vi "Laser_Control_1D.vi"() -> ()   [LabVIEW 2022 SP3]
uses:
  ADAM Client/Sub VIs/ADAM Controls/Update_scan_value.ctl
  Fibre_Flow_Mode.ctl
panel:
  out "GetMaxPower (mW)":dbl
  in  "stop":bool
  out "Loop No":i32
  in  "Power (mW)":dbl
  in  "Mode":T1
  out "error out":errorcluster
  in  "BSALaserCtrl.IBSALaser 2":refnum<k7>
  out "Status":string[](array[string])
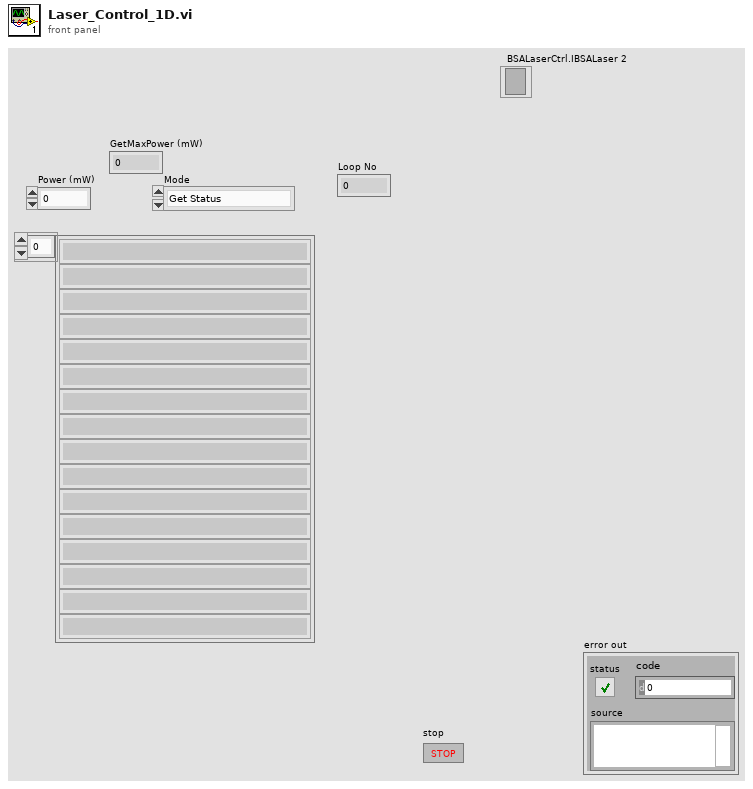
[diagram p1: front panel]
types:
  T1 = typedef "Fibre_Flow_Mode.ctl" = enum16{"Get Status", "Set Power", "Turn Laser On", "Turn Laser Off", "Shutter Open", "Shutter Closed", "Attenuated", "Disconnect"}
  T2 = typedef "Update_scan_value.ctl" = cluster{"Channel Name":string, "New Value":dbl, "!Auto_Off":bool}
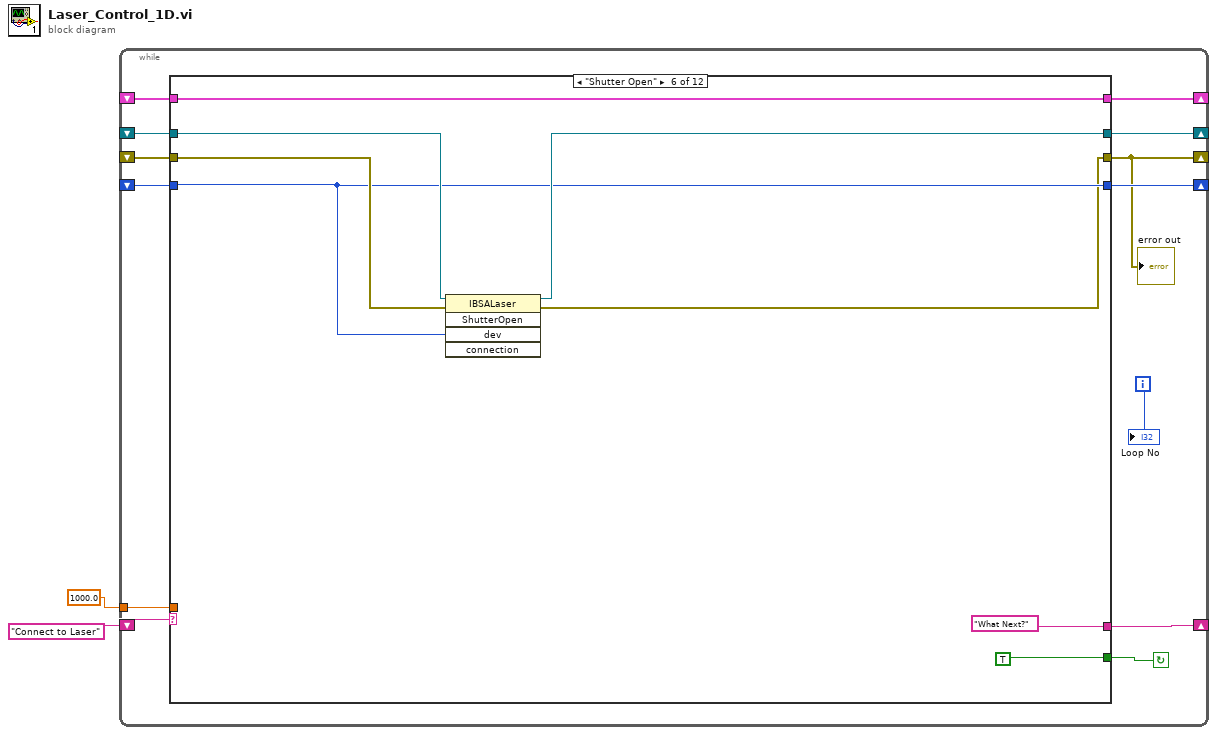
[diagram p0: block diagram]
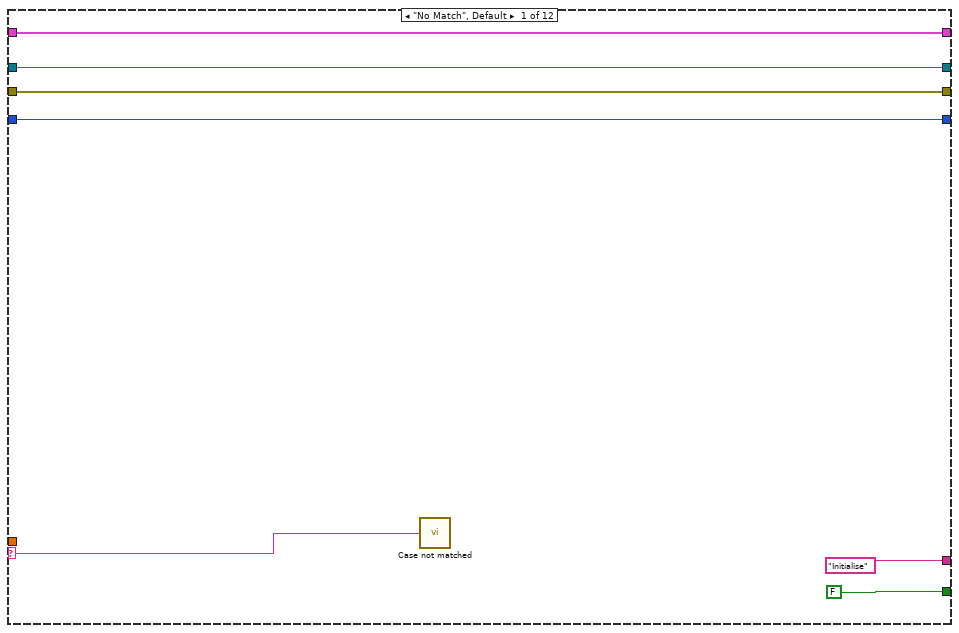
[diagram p2: hidden frame]
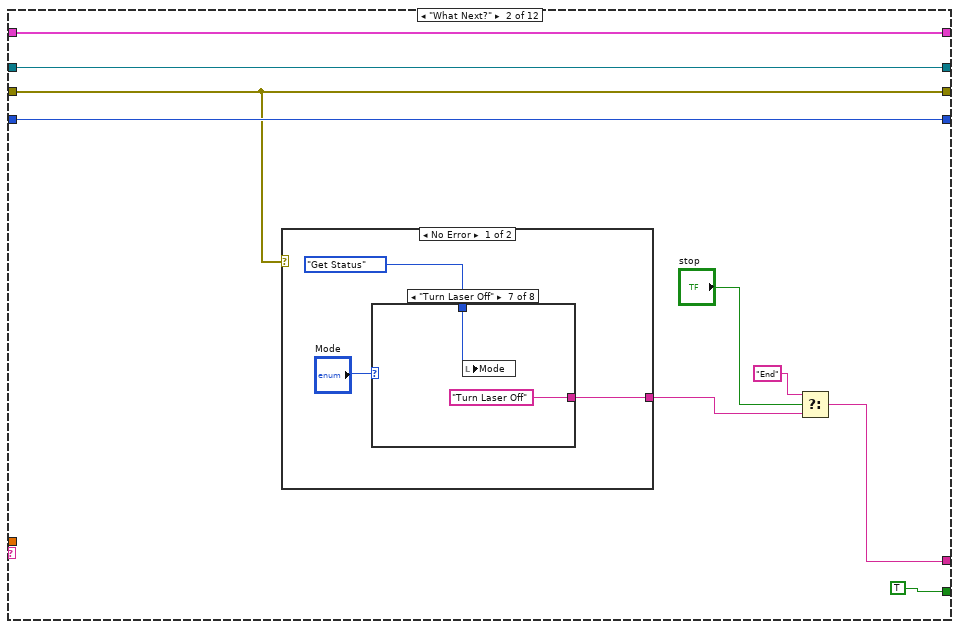
[diagram p3: hidden frame]
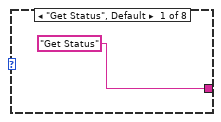
[diagram p4: hidden frame]
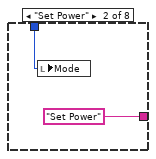
[diagram p5: hidden frame]
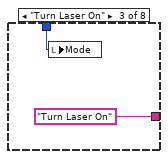
[diagram p6: hidden frame]
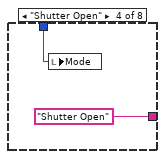
[diagram p7: hidden frame]
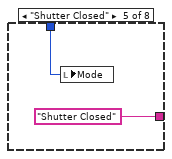
[diagram p8: hidden frame]
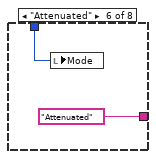
[diagram p9: hidden frame]
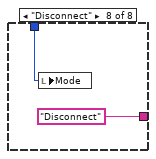
[diagram p10: hidden frame]
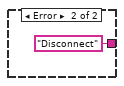
[diagram p11: hidden frame]
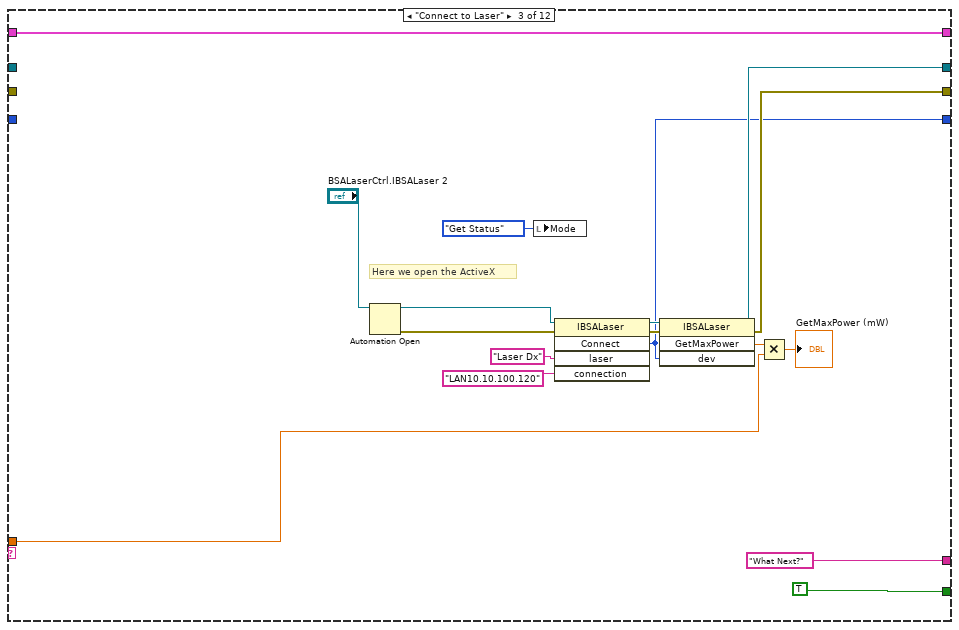
[diagram p12: hidden frame]
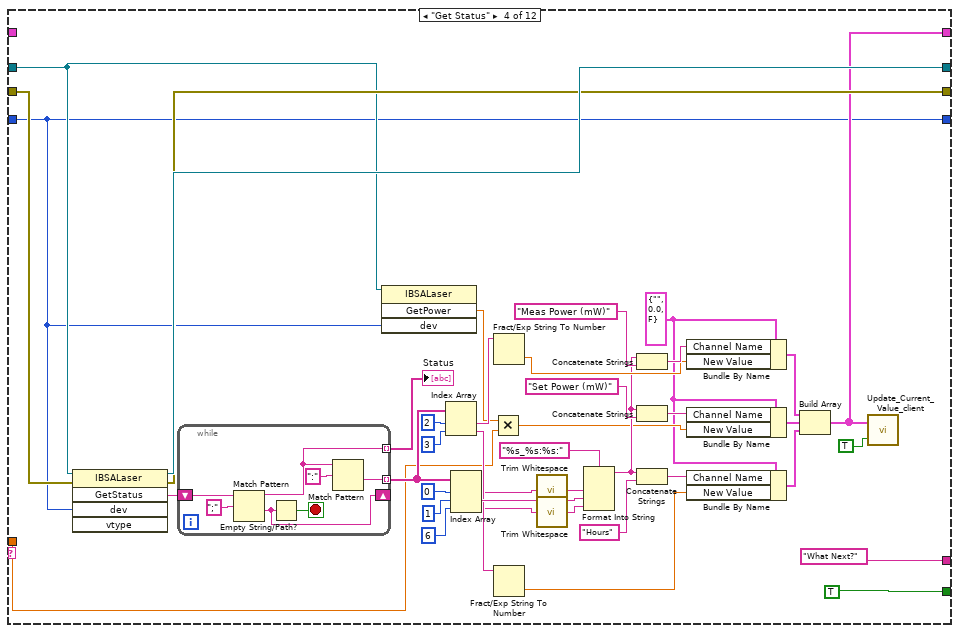
[diagram p13: hidden frame]
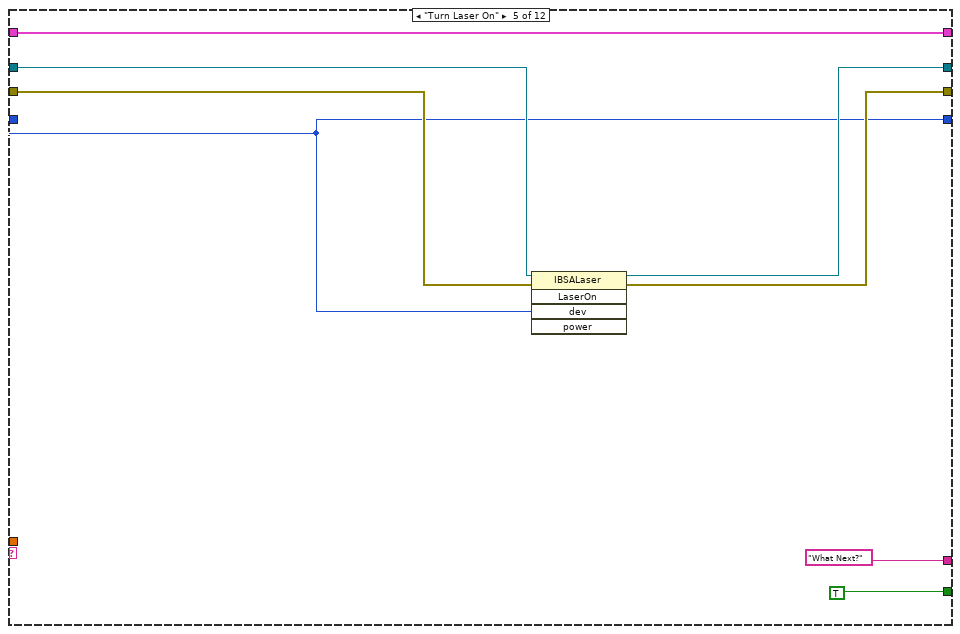
[diagram p14: hidden frame]
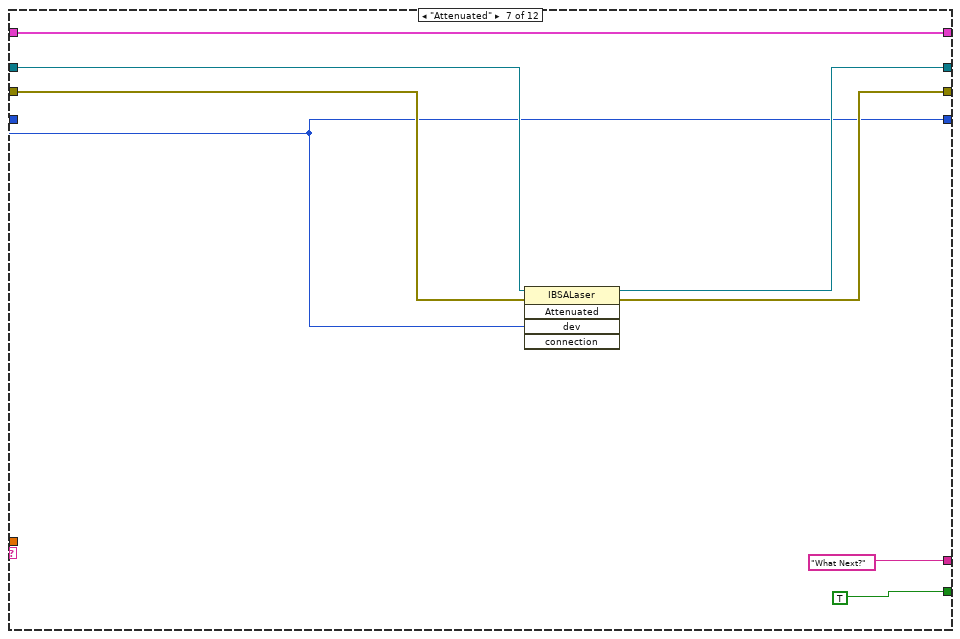
[diagram p15: hidden frame]
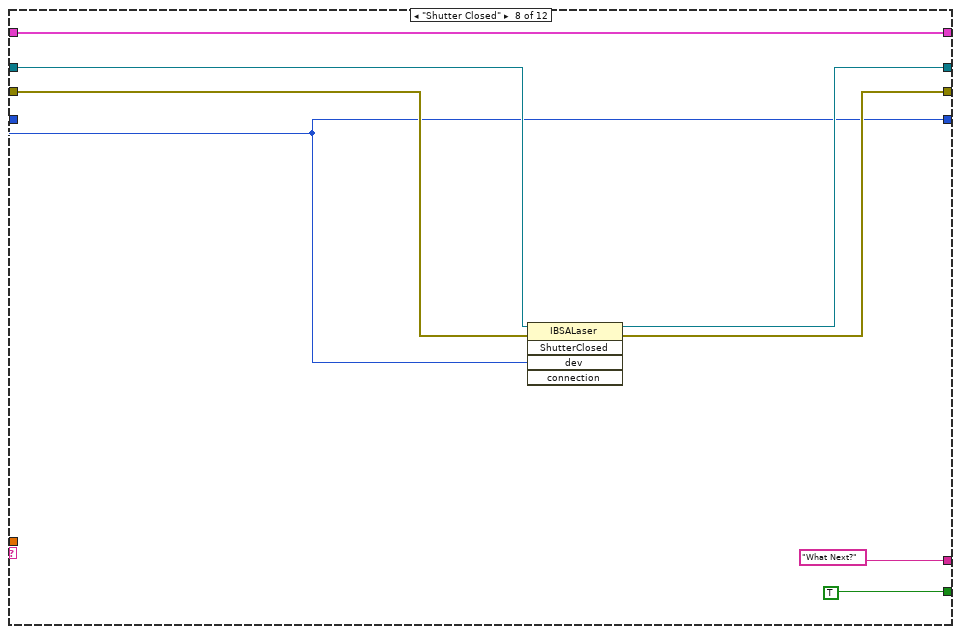
[diagram p16: hidden frame]
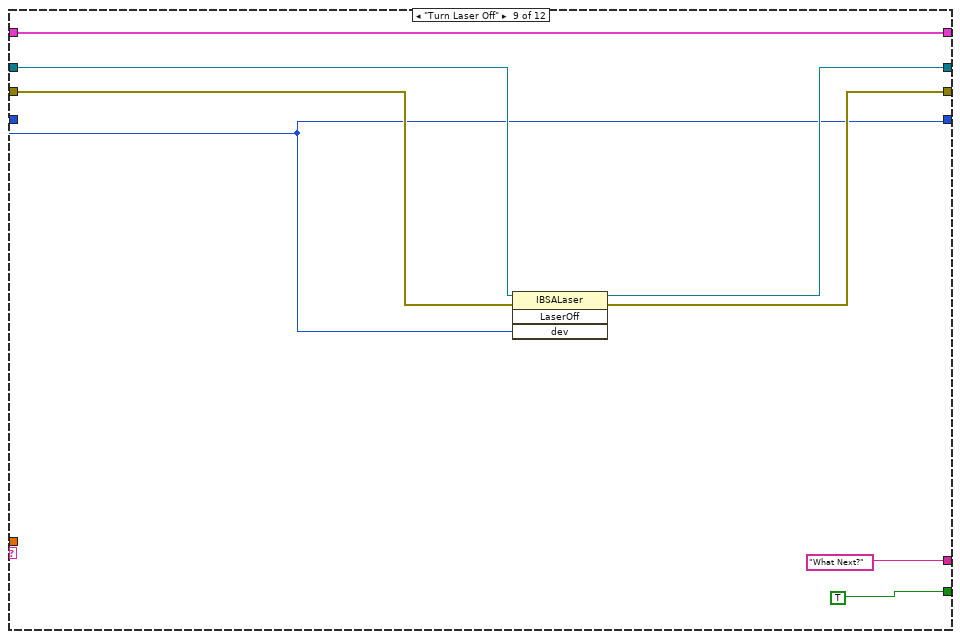
[diagram p17: hidden frame]
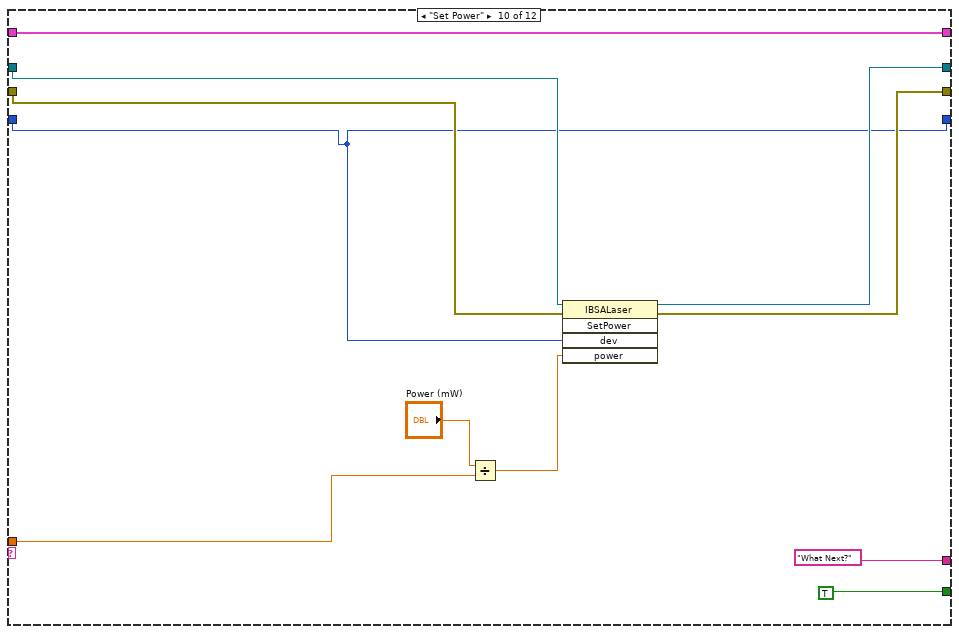
[diagram p18: hidden frame]
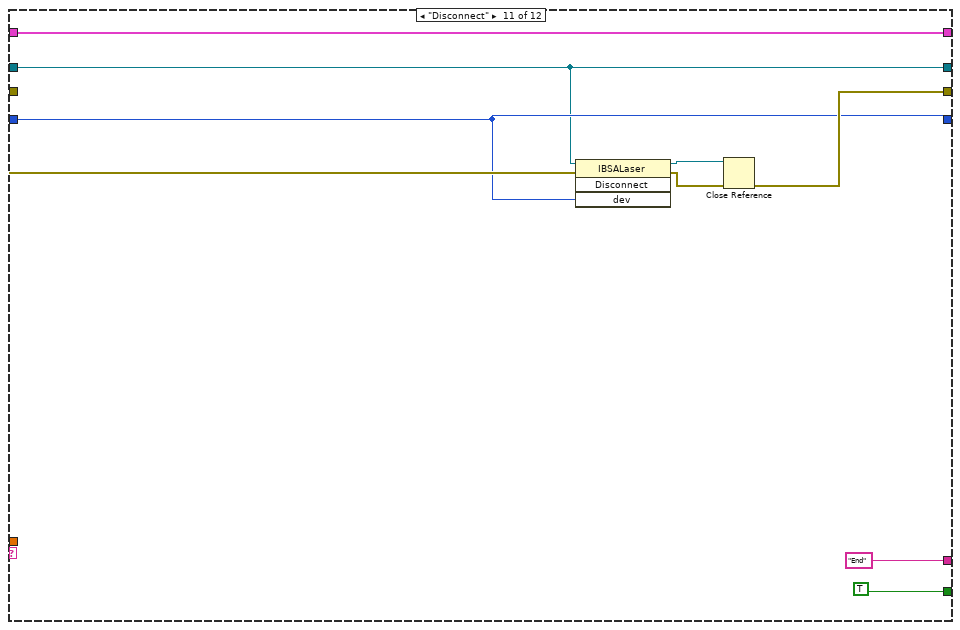
[diagram p19: hidden frame]
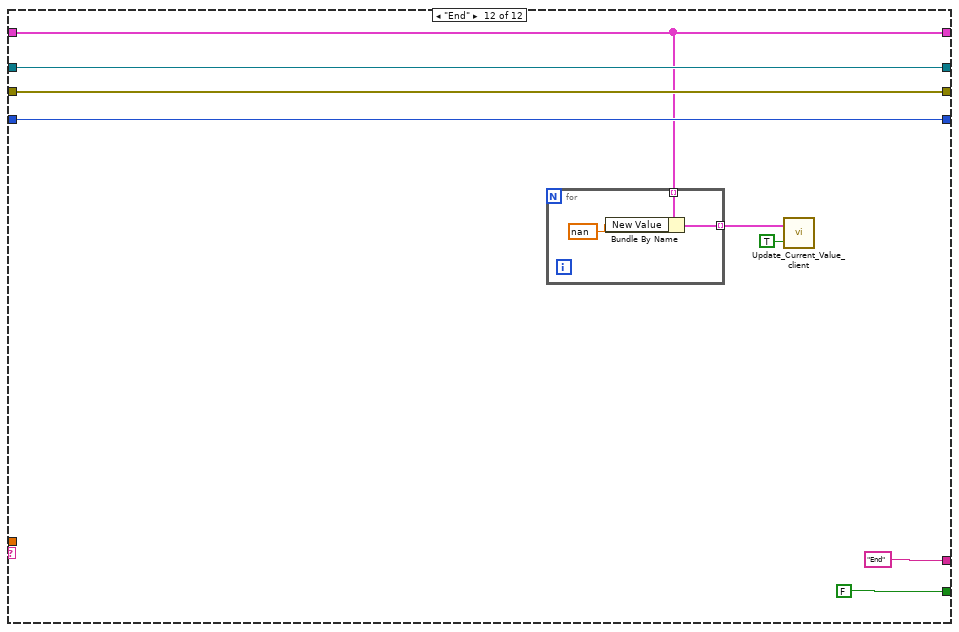
[diagram p20: hidden frame]
diagram:
  n1 = while {
    shift-left: "Connect to Laser" -> [w13]
    shift-right: [w14] -> _
    shift-right: [w12] -> _
    shift-left: _ -> [w10]
    shift-right: [w7] -> _
    shift-left: _ -> [w9]
    shift-right: [w11] -> _
    shift-left: _ -> [w8]
    shift-right: [w5] -> _
    shift-left: _ -> [w4]
    tunnel: 1000.0 ("y") -> [w3]
    i -> [w6]
    stop <- w15 continue-if-true
    n2 = case shown="\"Shutter Open\"" w13 {
      selector: w13 -> [w20 _ _ _ _ _ _ _ _ _ _ _]
      tunnel: [FALSE TRUE TRUE TRUE TRUE TRUE TRUE TRUE TRUE TRUE TRUE FALSE] -> w15
      tunnel: ["Initialise" w24 "What Next?" "What Next?" "What Next?" "What Next?" "What Next?" "What Next?" "What Next?" "What Next?" "End" "End"] -> w14
      tunnel: [w19 w31 w57 w104 w119 w127 w135 w143 w151 w162 w168 w180] -> w12
      tunnel: [w18 w29 w56 w103 w118 w124 w134 w142 w150 w161 w170 w179] -> w7
      tunnel: [w17 w30 w55 w78 w117 w126 w133 w141 w149 w160 w169 w181] -> w11
      tunnel: w10 -> [w19 w31 _ w79 w121 w129 w137 w145 w153 w164 w168 w180]
      tunnel: w9 -> [w18 w29 _ w105 w120 w128 w136 w144 w152 w163 w171 w179]
      tunnel: w8 -> [w17 w30 _ w78 w117 w126 w133 w141 w149 w160 w169 w181]
      tunnel: [w16 w28 w60 w80 w116 w125 w132 w140 w148 w159 w167 w177] -> w5
      tunnel: w4 -> [w16 w28 w60 _ w116 w125 w132 w140 w148 w159 w167 w177]
      tunnel: w3 -> [_ _ w52 w71 _ _ _ _ _ w157 _ _]
      frame "No Match", Default {
        n3 = call "Case not matched.vi"("Case Name not Matched"=w20) -> ()
      }
      frame "What Next?" {
        n4 = case shown="No Error" w29 {
          tunnel: [w33 "Disconnect"] -> w25
          frame No Error {
            n5 = case shown="\"Turn Laser Off\"" "Mode" {
              tunnel: ["Get Status" "Set Power" "Turn Laser On" "Shutter Open" "Shutter Closed" "Attenuated" "Turn Laser Off" "Disconnect"] -> w33
              tunnel: Fibre_Flow_Mode."Get Status" ("Mode") -> [_ w36 w38 w40 w42 w44 w46 w48]
              frame "Get Status", Default {
              }
              frame "Set Power" {
                n6 = local write "Mode"(w36) -> ()
              }
              frame "Turn Laser On" {
                n7 = local write "Mode"(w38) -> ()
              }
              frame "Shutter Open" {
                n8 = local write "Mode"(w40) -> ()
              }
              frame "Shutter Closed" {
                n9 = local write "Mode"(w42) -> ()
              }
              frame "Attenuated" {
                n10 = local write "Mode"(w44) -> ()
              }
              frame "Turn Laser Off" {
                n11 = local write "Mode"(w46) -> ()
              }
              frame "Disconnect" {
                n12 = local write "Mode"(w48) -> ()
              }
            }
          }
          frame Error {
          }
        }
        n13 = Select(t="End", s="stop", f=w25) -> (s? t:f=w24:string)
      }
      frame "Connect to Laser" {
        # "Here we open the ActiveX"
        n14 = Automation Open(Automation Refnum="BSALaserCtrl.IBSALaser 2") -> (Automation Refnum=w63:refnum<k7>, error out=w64:errorcluster)  [unwired: 3 in]
        n15 = local write "Mode"(Fibre_Flow_Mode."Get Status" ("Mode")) -> ()
        n16 = invoke class="IBSALaser" method="Connect"(reference=w63, error in=w64, "laser"="Laser Dx", "connection"="LAN10.10.100.120") -> (reference out=w59:refnum<k7>, error out=w58:errorcluster, "Connect"=w55:i64)  [unwired: 1 in, 2 out]
        n17 = invoke class="IBSALaser" method="GetMaxPower"(reference=w59, error in=w58, "dev"=w55) -> (reference out=w57:refnum<k7>, error out=w56:errorcluster, "GetMaxPower"=w54:dbl)  [unwired: 1 in, 1 out]
        n18 = Multiply(x=w54, y=w52) -> (x*y=→"GetMaxPower (mW)":dbl)
      }
      frame "Get Status" {
        w68 = T2 {"Channel Name"="", "New Value"=0.0, "!Auto_Off"=FALSE} ("Update Scan Value Cluster")
        n19 = invoke class="IBSALaser" method="GetStatus"(reference=w79, error in=w105, "dev"=w78) -> (reference out=w104:refnum<k7>, error out=w103:errorcluster, "GetStatus"=w106:string)  [unwired: 2 in, 2 out]
        n20 = while {
          shift-right: [w112] -> _
          shift-left: w106 -> [w114]
          tunnel: [w111] -> w102 mode=indexing
          tunnel: [w109] -> w93 mode=indexing
          stop <- w113 stop-if-true
          n21 = Match Pattern(string=w114, regular expression=";") -> (before substring=w111:string, after substring=w112:string)  [unwired: 1 in, 2 out]
          n22 = Empty String/Path?(string/path=w112) -> (empty?=w113:bool)
          n23 = Match Pattern(string=w111, regular expression=":") -> (after substring=w109:string)  [unwired: 1 in, 3 out]
        }
        "Status" <- w102
        n24 = invoke class="IBSALaser" method="GetPower"(reference=w79, "dev"=w78) -> ("GetPower"=w72:dbl)  [unwired: 2 in, 3 out]
        n25 = Index Array(array=w93, index #1=2 ("index"), index #2=3 ("index")) -> (element #1=w90:string, element #2=w88:string)
        n26 = Index Array(array=w93, index #1=0 ("index"), index #2=1 ("index"), index #3=6 ("index")) -> (element #1=w82:string, element #2=w98:string, element #3=w84:string)
        n27 = Multiply(x=w72, y=w71) -> (x*y=w70:dbl)
        n28 = Fract/Exp String To Number(string=w90) -> (number=w89:dbl)  [unwired: 3 in, 1 out]
        n29 = Fract/Exp String To Number(string=w88) -> (number=w75:dbl)  [unwired: 3 in, 1 out]
        n30 = call <vilib>:"Trim Whitespace.vi"("string"=w82) -> ("trimmed string"=w81:string)  [unwired: 1 in]
        n31 = call <vilib>:"Trim Whitespace.vi"("string"=w84) -> ("trimmed string"=w83:string)  [unwired: 1 in]
        n32 = Format Into String(format string="%s_%s:%s:", w81, w98, w83) -> (resulting string=w76:string)  [unwired: 2 in, 1 out]
        n33 = Concatenate Strings(w76, "Meas Power (mW)" ("string")) -> (w94:string)
        n34 = Concatenate Strings(w76, "Set Power (mW)" ("string")) -> (w73:string)
        n35 = Concatenate Strings(w76, "Hours" ("string")) -> (w74:string)
        n36 = Bundle By Name(cluster=w68, "Channel Name"=w94, "New Value"=w89) -> (w87:T2)
        n37 = Bundle By Name(cluster=w68, "Channel Name"=w73, "New Value"=w70) -> (w86:T2)
        n38 = Bundle By Name(cluster=w68, "Channel Name"=w74, "New Value"=w75) -> (w69:T2)
        n39 = Build Array(w87, w86, w69) -> (w80:T2[])
        n40 = call "Update_Current_Value_client.vi"("Don't Bother with check?"=TRUE, "Update array in"=w80) -> ()
      }
      frame "Turn Laser On" {
        n41 = invoke class="IBSALaser" method="LaserOn"(reference=w121, error in=w120, "dev"=w117) -> (reference out=w119:refnum<k7>, error out=w118:errorcluster)  [unwired: 2 in, 3 out]
      }
      frame "Shutter Open" {
        n42 = invoke class="IBSALaser" method="ShutterOpen"(reference=w129, error in=w128, "dev"=w126) -> (reference out=w127:refnum<k7>, error out=w124:errorcluster)  [unwired: 2 in, 3 out]
      }
      frame "Attenuated" {
        n43 = invoke class="IBSALaser" method="Attenuated"(reference=w137, error in=w136, "dev"=w133) -> (reference out=w135:refnum<k7>, error out=w134:errorcluster)  [unwired: 2 in, 3 out]
      }
      frame "Shutter Closed" {
        n44 = invoke class="IBSALaser" method="ShutterClosed"(reference=w145, error in=w144, "dev"=w141) -> (reference out=w143:refnum<k7>, error out=w142:errorcluster)  [unwired: 2 in, 3 out]
      }
      frame "Turn Laser Off" {
        n45 = invoke class="IBSALaser" method="LaserOff"(reference=w153, error in=w152, "dev"=w149) -> (reference out=w151:refnum<k7>, error out=w150:errorcluster)  [unwired: 1 in, 2 out]
      }
      frame "Set Power" {
        n46 = Divide(x="Power (mW)", y=w157) -> (x/y=w156:dbl)
        n47 = invoke class="IBSALaser" method="SetPower"(reference=w164, error in=w163, "dev"=w160, "power"=w156) -> (reference out=w162:refnum<k7>, error out=w161:errorcluster)  [unwired: 1 in, 3 out]
      }
      frame "Disconnect" {
        n48 = invoke class="IBSALaser" method="Disconnect"(reference=w168, error in=w171, "dev"=w169) -> (reference out=w172:refnum<k7>, error out=w173:errorcluster)  [unwired: 1 in, 2 out]
        n49 = Close Reference(reference=w172, error in (no error)=w173) -> (error out=w170:errorcluster)
      }
      frame "End" {
        n50 = for {
          tunnel: [w185] -> w176 mode=indexing
          tunnel: w177 -> [w184] mode=indexing
          n51 = Bundle By Name(cluster=w184, "New Value"=nan) -> (w185:T2)
        }
        n52 = call "Update_Current_Value_client.vi"("Don't Bother with check?"=TRUE, "Update array in"=w176) -> ()
      }
    }
    "error out" <- w7
    "Loop No" <- w6
  }
